vi "Mark_Clicked_Selected.vi"(5 "Coords":T2, 6 "error in (no error)":errorcluster, 7 "EventType":T1, 8 "Id":string, 9 "EpiWrapper in":refnum<class "EpiWrapper.lvclass">) -> (0 "error out":errorcluster, 3 "EpiWrapper out":refnum<class "EpiWrapper.lvclass">)   [LabVIEW 2012, in "EpiWrapper.lvclass"]
uses:
  EpiWrapper.lvclass
  <vilib>/Utility/miscctls.llb/LVPoint32TypeDef.ctl
  Controls/MapEventType.ctl
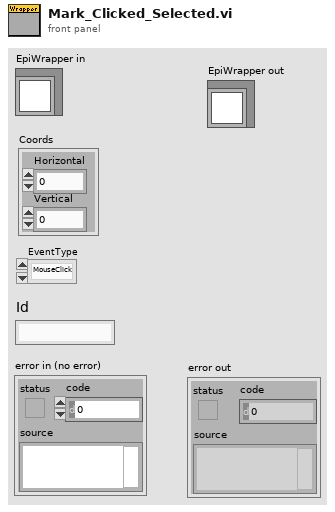
[diagram p1: front panel]
types:
  T1 = typedef "MapEventType.ctl" = enum16{"MouseClick", "DropDown"}
  T2 = typedef "LVPoint32TypeDef.ctl" = cluster{"Horizontal":i32, "Vertical":i32}
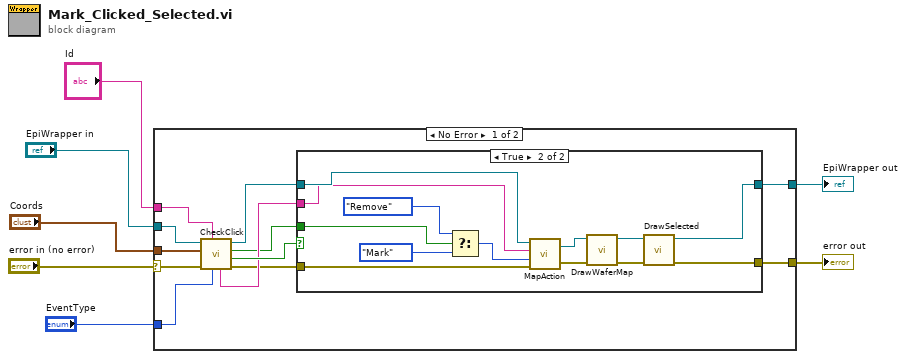
[diagram p0: block diagram]
diagram:
  n1 = case shown="No Error" "error in (no error)" {
    selector: "error in (no error)" -> [w16 w36]
    tunnel: [w8 w36] -> w6
    tunnel: [w9 w35] -> w4
    tunnel: "EpiWrapper in" -> [w17 w35]
    tunnel: "Id" -> [w13 _]
    tunnel: "Coords" -> [w19 _]
    tunnel: "EventType" -> [w18 _]
    frame No Error {
      n2 = call-dynamic "CheckClick.vi"("Enum"=w18, "Pad"=w13, "error in (no error)"=w16, "Coords"=w19, "EpiWrapper in"=w17) -> ("error out"=w10:errorcluster, "OnPad?"=w15:bool, "Selected?"=w11:bool, "EpiWrapper out"=w12:refnum<class "EpiWrapper.lvclass">, "Id"=w14:string)  [unwired: 2 in]
      n3 = case shown="True" w15 {
        tunnel: w14 -> [_ w25]
        tunnel: w12 -> [w21 w30]
        tunnel: w11 -> [_ w27]
        tunnel: w10 -> [w20 w24]
        tunnel: [w21 w23] -> w9
        tunnel: [w20 w22] -> w8
        frame False {
        }
        frame True {
          n4 = Select(t=enum16{"Remove", "Mark", "Clear All"}."Remove" ("Enum"), s=w27, f=enum16{"Remove", "Mark", "Clear All"}."Mark" ("Enum")) -> (s? t:f=w26:enum16{"Remove", "Mark", "Clear All"})
          n5 = call-dynamic "MapAction.vi"("error in (no error)"=w24, "Action"=w26, "Id"=w25, "EpiWrapper in"=w30) -> ("error out"=w33:errorcluster, "EpiWrapper out"=w32:refnum<class "EpiWrapper.lvclass">)
          n6 = call-dynamic "DrawWaferMap.vi"("error in (no error)"=w33, "EpiWrapper in"=w32) -> ("error out"=w34:errorcluster, "EpiWrapper out"=w31:refnum<class "EpiWrapper.lvclass">)  [unwired: 8 in]
          n7 = call-dynamic "DrawSelected.vi"("error in (no error)"=w34, "EpiWrapper in"=w31) -> ("error out"=w22:errorcluster, "EpiWrapper out"=w23:refnum<class "EpiWrapper.lvclass">)  [unwired: 8 in]
        }
      }
    }
    frame Error {
    }
  }
  "error out" <- w6
  "EpiWrapper out" <- w4
